vi "Read Filter settings.vi"(8 "error in (no error)":errorcluster, 11 "Realsense Cam in":refnum<class "Realsense Cam.lvclass">) -> (0 "error out":errorcluster, 2 "Filter settings":T1={"Decimation Scale (1-10)"=3, "Spatial Alpha\n(0-1)"=0.6, "Spatial Delta \n(1/32 disp)"=8, "Temporal Alpha\n(0-1)"=0.4, "Temporal Delta\n(1/32 disp)"=20, "Persistence (0= none, 8=max)"=0, "spatial holefill radius\n(0 disable, 5 max) "=0, "spatial iteration\n(2=default)"=2} {"spatial iteration\n(2=default)" min=1 max=10; "Decimation Scale (1-10)" min=1 max=10; "Spatial Alpha\n(0-1)" min=0 max=1 format="%_2g"; "Spatial Delta \n(1/32 disp)" min=1; "Temporal Alpha\n(0-1)" min=0 max=1 format="%_2g"; "Temporal Delta\n(1/32 disp)" min=1; "Persistence (0= none, 8=max)" max=8; "spatial holefill radius\n(0 disable, 5 max)" max=6}, 3 "Realsense Cam out":refnum<class "Realsense Cam.lvclass">)   [LabVIEW 2018, in "Realsense Cam.lvclass"]
uses:
  Realsense Cam.lvclass
  Realsense Cam.lvclass/Realsense Cam.ctl
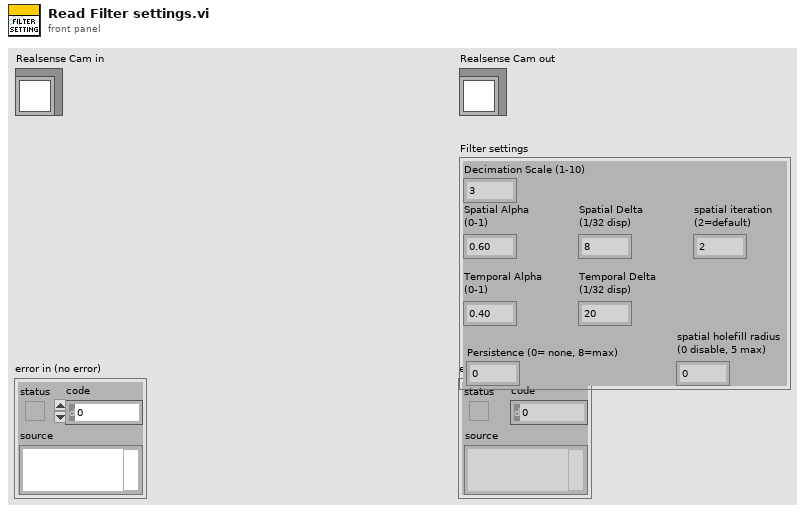
[diagram p1: front panel]
types:
  T1 = cluster{"Decimation Scale (1-10)":u8, "Spatial Alpha\n(0-1)":sgl, "Spatial Delta \n(1/32 disp)":u16, "Temporal Alpha\n(0-1)":sgl, "Temporal Delta\n(1/32 disp)":u16, "Persistence (0= none, 8=max)":u8, "spatial holefill radius\n(0 disable, 5 max) ":u8, "spatial iteration\n(2=default)":u8}
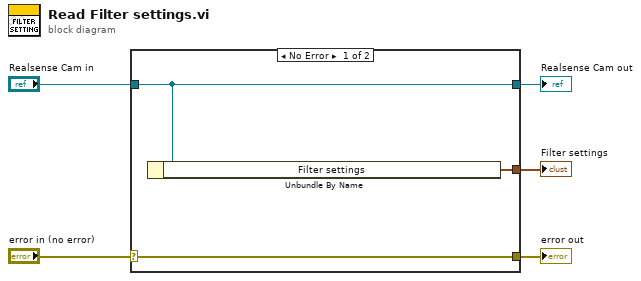
[diagram p0: block diagram]
diagram:
  n1 = case shown="No Error" "error in (no error)" {
    selector: "error in (no error)" -> [w8 w9]
    tunnel: [w8 w9] -> w4
    tunnel: [w7 w10] -> w2
    tunnel: "Realsense Cam in" -> [w7 w10]
    tunnel: [w6 _] -> w1
    frame No Error {
      n2 = Unbundle By Name(w7) -> ("Filter settings"=w6:T1)
    }
    frame Error {
    }
  }
  "error out" <- w4
  "Realsense Cam out" <- w2
  "Filter settings" <- w1
